vi "Test Method Done.vi"(8 "error in (no error)":errorcluster, 11 "Slave Test Runner in":refnum<class "Slave Test Runner.lvclass">) -> (0 "error out":errorcluster, 3 "Slave Test Runner out":refnum<class "Slave Test Runner.lvclass">)   [LabVIEW 2020, in "Slave Test Runner.lvclass"]
uses:
  Slave Test Runner.lvclass
  Slave Test Runner.lvclass/Slave Test Runner.ctl
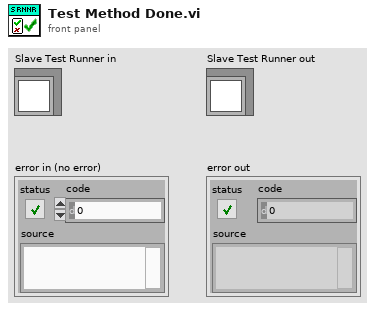
[diagram p1: front panel]
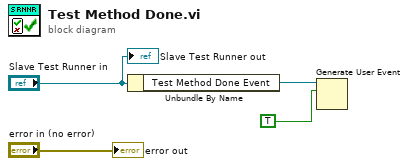
[diagram p0: block diagram]
diagram:
  n1 = Unbundle By Name("Slave Test Runner in") -> ("Test Method Done Event"=w3:refnum<user-event>)
  n2 = Generate User Event(user event=w3, event data cluster=TRUE ("event data")) -> ()  [unwired: 2 in, 2 out]
  "Slave Test Runner out" <- "Slave Test Runner in"
  "error out" <- "error in (no error)"
